vi "List Status in Registry.vi"(0 "BroadcastRegistry in":refnum<class "BroadcastRegistry.lvclass">) -> (4 "BroadcastRegistry out":refnum<class "BroadcastRegistry.lvclass">, 6 "Status":string[](array[string]))   [LabVIEW 2020, in "Communicable State Machine.lvlib" / "BroadcastRegistry.lvclass"]
uses:
  BroadcastRegistry.lvclass
  BroadcastRegistry.lvclass/BroadcastRegistry.ctl
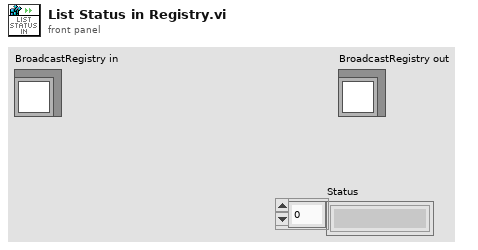
[diagram p1: front panel]
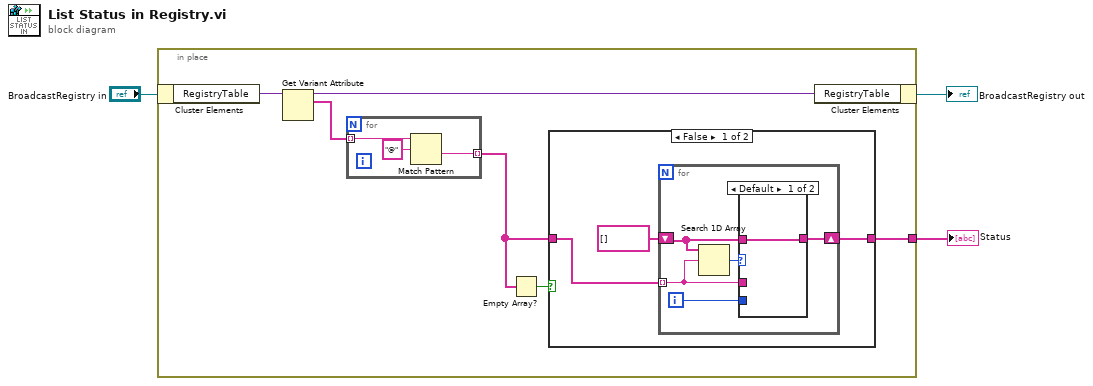
[diagram p0: block diagram]
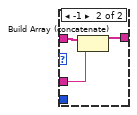
[diagram p2: hidden frame]
diagram:
  n1 = in-place {
    in-place-border: [w9] -> w1
    n2 = in-place-cluster #1("BroadcastRegistry in") -> ("RegistryTable"=w8:variant)
    n3 = Get Variant Attribute(Variant=w8) -> (duplicate Variant=w7:variant, names=w5:string[])  [unwired: 3 in, 2 out]
    n4 = for {
      tunnel: w5 -> [w12] mode=indexing
      tunnel: [w10] -> w4 mode=indexing
      n5 = Match Pattern(string=w12, regular expression="@") -> (after substring=w10:string)  [unwired: 1 in, 3 out]
    }
    n6 = Empty Array?(array=w4) -> (empty?=w6:bool)
    n7 = case shown="False" w6 {
      tunnel: w4 -> [w14 w25]
      tunnel: [w15 w25] -> w9
      frame False {
        n8 = for {
          tunnel: w14 -> [w19] mode=indexing
          shift-right: [w18] -> w15
          shift-left: string[] [] -> [w16]
          i -> [w17]
          n9 = Search 1D Array(1D array=w16, element=w19) -> (index of element=w20:i32)  [unwired: 1 in]
          n10 = case shown="Default" w20 {
            tunnel: w19 -> [_ w24]
            tunnel: [w21 w23] -> w18
            tunnel: w17 -> [_ _]
            tunnel: w16 -> [w21 w22]
            frame Default {
            }
            frame -1 {
              n11 = Build Array (concatenate)(w22, w24) -> (w23:string[])
            }
          }
        }
      }
      frame True {
      }
    }
    n12 = in-place-cluster #1("RegistryTable"=w7) -> (→"BroadcastRegistry out":refnum<class "BroadcastRegistry.lvclass">)
  }
  "Status" <- w1
